vi "Compass.vi"(6 "Stop Program":bool, 8 "East or West":string, 9 "Longitude":dbl format="%_16g", 10 "North or South":string, 11 "Latitude":dbl format="%_16g") -> (3 "Compass":dbl(xcontrol))   [LabVIEW 2011]
uses:
  <vilib>/robotics/Controls/Compass Indicator/Compass Indicator.xctl
  <vilib>/express/express arith-compare/Formula/XNode/ExpressFormulaBlockNode.xnode
panel:
  out "Compass Lat Array":dbl[](array[numeric])
  out "Compass Long Array":dbl[](array[numeric])
  out "Compass N/S Array":string[](array[string])
  out "Compass E/W Array":string[](array[string])
  out "Compass Long":dbl
  out "Compass Lat":dbl
  out "Compass E/W":string
  out "Compass N/S":string
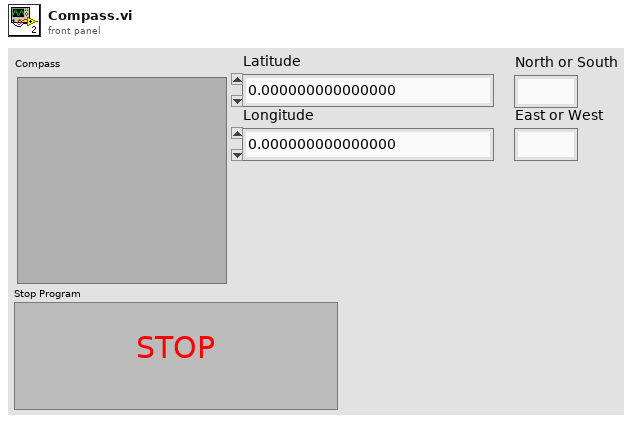
[diagram p1: front panel]
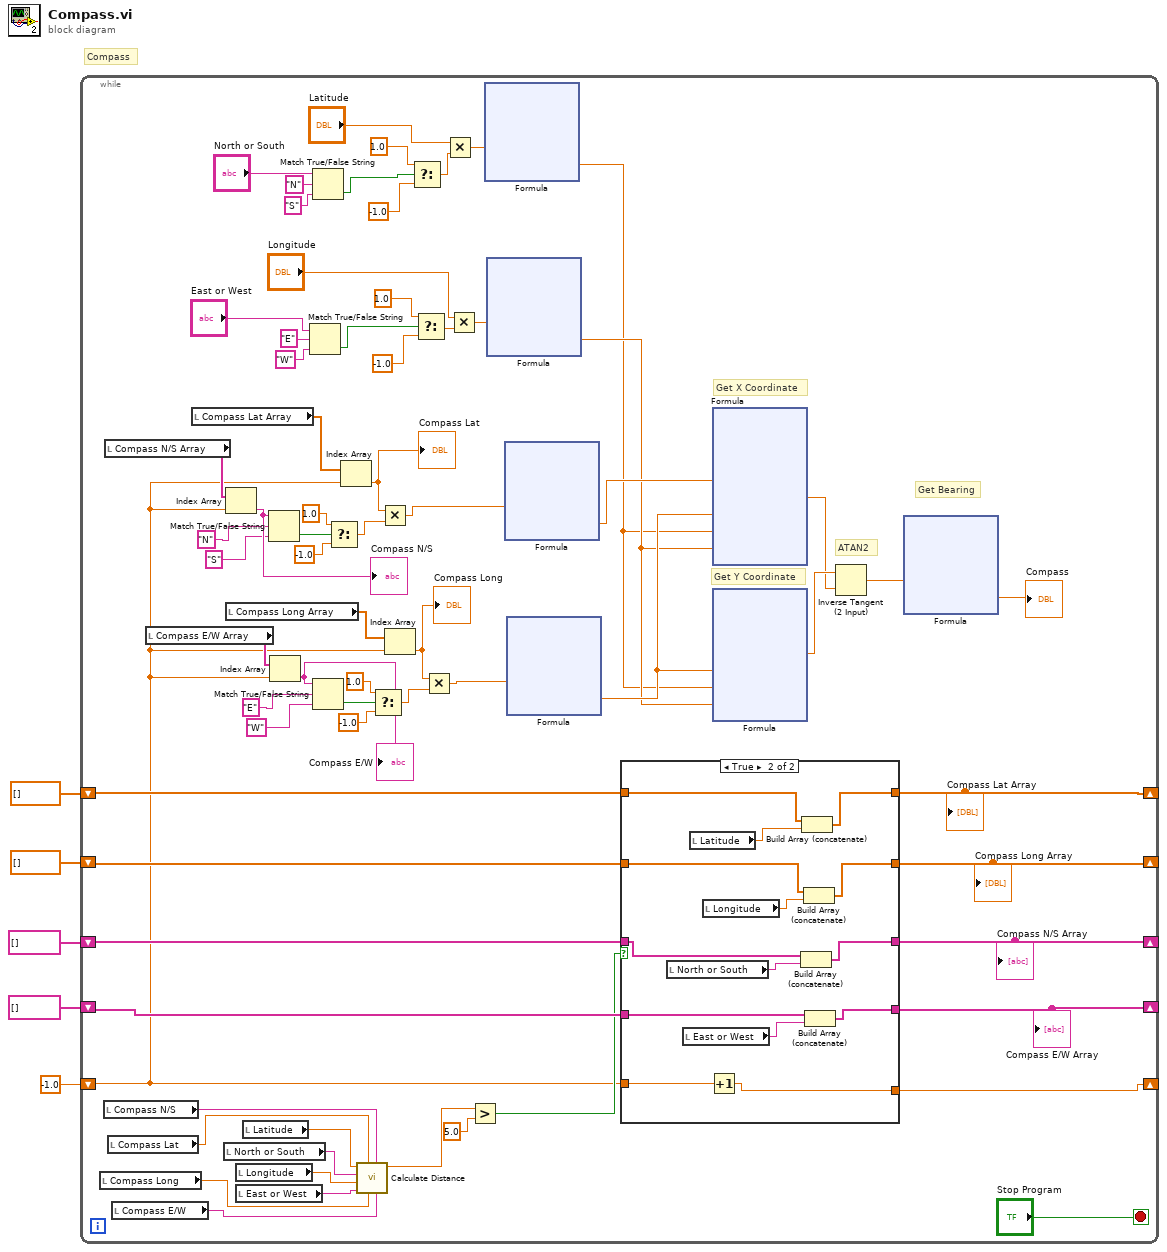
[diagram p0: block diagram]
diagram:
  # "Compass"
  n1 = while {
    shift-right: [w71] -> _
    shift-left: dbl[] [] -> [w72]
    shift-right: [w70] -> _
    shift-left: dbl[] [] -> [w73]
    shift-right: [w69] -> _
    shift-left: string[] [] -> [w74]
    shift-right: [w68] -> _
    shift-left: string[] [] -> [w75]
    shift-right: [w12] -> _
    shift-left: -1.0 -> [w11]
    stop <- "Stop Program" stop-if-true
    # "Get X Coordinate"
    # "Get Bearing"
    # "ATAN2"
    # "Get Y Coordinate"
    n2 = local read "Compass Long"() -> (w17:dbl)
    n3 = local read "Compass N/S"() -> (w18:string)
    n4 = local read "Compass N/S Array"() -> (w66:string[])
    n5 = local read "Compass Lat"() -> (w19:dbl)
    n6 = local read "Compass E/W"() -> (w16:string)
    n7 = local read "Compass E/W Array"() -> (w63:string[])
    n8 = local read "Compass Lat Array"() -> (w65:dbl[])
    n9 = local read "North or South"() -> (w22:string)
    n10 = Index Array(array=w66, index=w11) -> (element=w57:string)
    "Compass N/S" <- w57
    n11 = local read "Compass Long Array"() -> (w64:dbl[])
    n12 = local read "Longitude"() -> (w21:dbl)
    n13 = local read "East or West"() -> (w20:string)
    n14 = local read "Latitude"() -> (w23:dbl)
    n15 = Match True/False String(2:"S" ("false string"), 3:"N" ("true string"), 4:w57) -> (0:w52:bool)  [unwired: 1 out]
    n16 = Index Array(array=w63, index=w11) -> (element=w58:string)
    "Compass E/W" <- w58
    n17 = Match True/False String(2:"W" ("false string"), 3:"E" ("true string"), 4:"East or West") -> (0:w33:bool)  [unwired: 1 out]
    n18 = Match True/False String(2:"S" ("false string"), 3:"N" ("true string"), 4:"North or South") -> (0:w32:bool)  [unwired: 1 out]
    n19 = Match True/False String(2:"W" ("false string"), 3:"E" ("true string"), 4:w58) -> (0:w46:bool)  [unwired: 1 out]
    n20 = Select(t=1.0, s=w52, f=-1.0) -> (s? t:f=w53:dbl)
    n21 = Index Array(array=w65, index=w11) -> (element=w61:dbl)
    "Compass Lat" <- w61
    n22 = call "Calculate Distance.vi"("Prime Meridian Destination Direction"=w16, "Equator Destination Direction"=w18, "Destination Longitude"=w17, "Destination Latitude"=w19, "East or West"=w20, "Longitude"=w21, "North or South"=w22, "Latitude"=w23) -> ("Distance (ft)"=w15:dbl)  [unwired: 3 in]
    n23 = Select(t=1.0, s=w46, f=-1.0) -> (s? t:f=w47:dbl)
    n24 = Multiply(x=w61, y=w53) -> (x*y=w62:dbl)
    n25 = Index Array(array=w64, index=w11) -> (element=w59:dbl)
    "Compass Long" <- w59
    n26 = Select(t=1.0, s=w32, f=-1.0) -> (s? t:f=w27:dbl)
    n27 = Select(t=1.0, s=w33, f=-1.0) -> (s? t:f=w26:dbl)
    n28 = Multiply(x=w59, y=w47) -> (x*y=w60:dbl)
    n29 = Multiply(x="Latitude", y=w27) -> (x*y=w38:dbl)
    n30 = Multiply(x="Longitude", y=w26) -> (x*y=w39:dbl)
    n31 = Greater?(x=w15, y=5.0) -> (0:w13:bool)
    n32 = xnode "Formula"("Dlat1"=w38) -> ("Result"=w24:dbl)  [unwired: 1 in, 1 out]
    n33 = xnode "Formula"("Dlong1"=w39) -> ("Result"=w25:dbl)  [unwired: 1 in, 1 out]
    n34 = xnode "Formula"("Dlat1"=w62) -> ("Result"=w43:dbl)  [unwired: 1 in, 1 out]
    n35 = xnode "Formula"("Dlong1"=w60) -> ("Result"=w44:dbl)  [unwired: 1 in, 1 out]
    n36 = case shown="True" w13 {
      tunnel: w72 -> [w146 w156]
      tunnel: w73 -> [w145 w155]
      tunnel: w74 -> [w144 w154]
      tunnel: w75 -> [w143 w153]
      tunnel: [w146 w152] -> w71
      tunnel: [w145 w151] -> w70
      tunnel: [w144 w150] -> w69
      tunnel: [w143 w149] -> w68
      tunnel: w11 -> [w142 w148]
      tunnel: [w142 w147] -> w12
      frame False {
      }
      frame True {
        n37 = local read "North or South"() -> (w160:string)
        n38 = local read "East or West"() -> (w159:string)
        n39 = local read "Latitude"() -> (w157:dbl)
        n40 = local read "Longitude"() -> (w158:dbl)
        n41 = Increment(x=w148) -> (x+1=w147:dbl)
        n42 = Build Array (concatenate)(w154, w160) -> (w150:string[])
        n43 = Build Array (concatenate)(w156, w157) -> (w152:dbl[])
        n44 = Build Array (concatenate)(w155, w158) -> (w151:dbl[])
        n45 = Build Array (concatenate)(w153, w159) -> (w149:string[])
      }
    }
    "Compass Lat Array" <- w71
    "Compass Long Array" <- w70
    "Compass N/S Array" <- w69
    "Compass E/W Array" <- w68
    n46 = xnode "Formula"("PreLat"=w43, "PreLong"=w44, "CurLat"=w24, "CurLong"=w25) -> ("Result"=w41:dbl)  [unwired: 1 in, 1 out]
    n47 = xnode "Formula"("PreLong"=w44, "CurLat"=w24, "CurLong"=w25) -> ("Result"=w42:dbl)  [unwired: 1 in, 1 out]
    n48 = Inverse Tangent (2 Input)(1:w41, 2:w42) -> (0:w40:dbl)
    n49 = xnode "Formula"("rad"=w40) -> ("Result"=→"Compass":dbl)  [unwired: 1 in, 1 out]
  }
